vi "CurrentConditionDisplay_Create.vi"(0 "reference in":refnum<class "CurrentConditionDisplay.lvclass">, 5 "error in (no error)":errorcluster) -> (14 "reference out":refnum<class "CurrentConditionDisplay.lvclass">, 19 "error out":errorcluster)   [LabVIEW 2020, in "CurrentConditionDisplay.lvclass"]
uses:
  CurrentConditionDisplay.lvclass
  C:/Projects/OpenGDS_DesignPatterns/Observer1_WheaterStation/Observer_class/Observer.lvclass
  Observer_class/Observer.lvclass
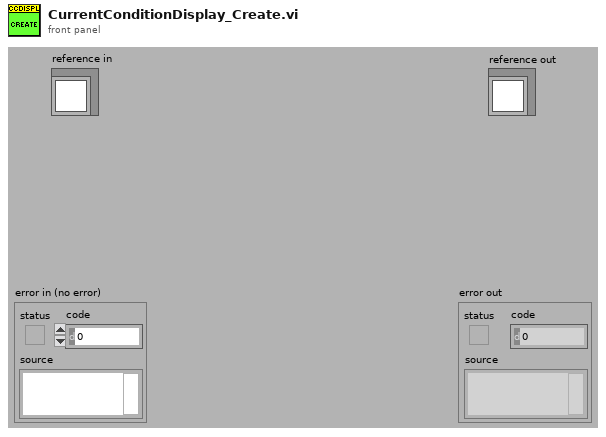
[diagram p1: front panel]
types:
  T1 = typedef "CurrentConditionDisplay.lvclass/ObjectAttributes.ctl" = cluster{"WeatherData":T2}
  T2 = typedef "WeatherData.ctl" = cluster{"Temperature C":dbl, "Humid %":dbl, "Pressure":dbl, "Forecast":string}
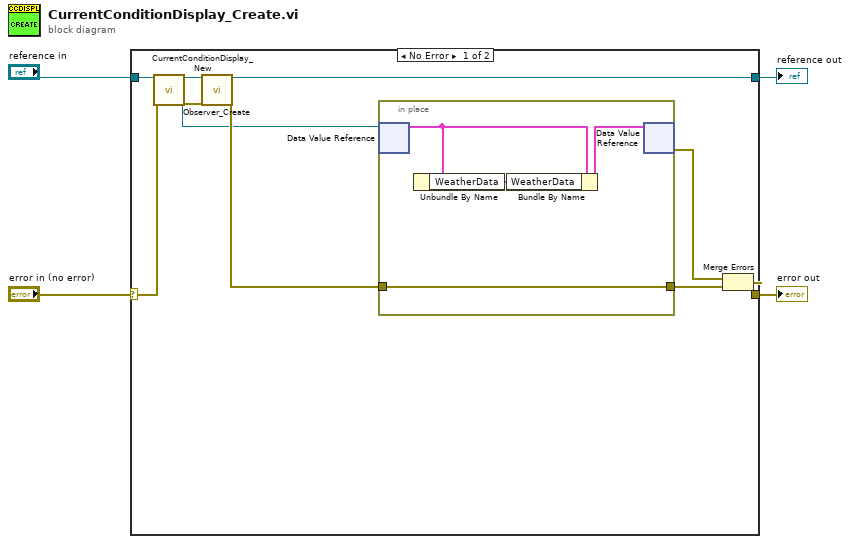
[diagram p0: block diagram]
diagram:
  n1 = case shown="No Error" "error in (no error)" {
    selector: "error in (no error)" -> [w8 w20]
    tunnel: [w12 w20] -> w3
    tunnel: "reference in" -> [w9 w19]
    tunnel: [w14 w19] -> w1
    frame No Error {
      n2 = call "CurrentConditionDisplay_New.vi"("reference in"=w9, "error in (no error)"=w8) -> ("reference out"=w7:refnum<class "CurrentConditionDisplay.lvclass">, "DVRRefOut"=w5:refnum<data-value>, "error out"=w6:errorcluster)  [unwired: 14 in, 1 out]
      n3 = call "Observer_Create.vi"("reference in"=w7, "error in (no error)"=w6) -> ("reference out"=w14:refnum<class "CurrentConditionDisplay.lvclass">, "error out"=w11:errorcluster)  [unwired: 16 in]
      n4 = in-place {
        in-place-border: w11 -> [w15]
        in-place-border: [w15] -> w10
        n5 = in-place-dvr #1(w5) -> (w17:T1)  [unwired: 1 out]
        n6 = Unbundle By Name(w17) -> ("WeatherData"=w16:T2)
        n7 = Bundle By Name(cluster=w17, "WeatherData"=w16) -> (w18:T1)
        n8 = in-place-dvr #1(w18) -> (w13:errorcluster)  [unwired: 1 out]
      }
      n9 = Merge Errors(w13, w10) -> (w12:errorcluster)
    }
    frame Error {
    }
  }
  "error out" <- w3
  "reference out" <- w1
